vi "4.7.vi"() -> ()   [LabVIEW 2017]
panel:
  out "猜测次数":dbl
  out "随机的数":dbl
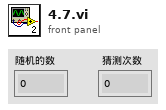
[diagram p1: front panel]
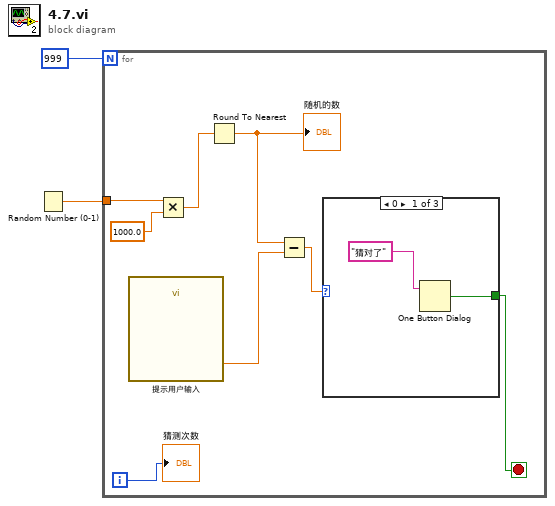
[diagram p0: block diagram]
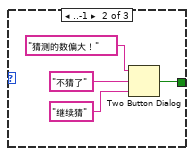
[diagram p2: hidden frame]
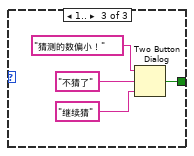
[diagram p3: hidden frame]
diagram:
  n1 = Random Number (0-1)() -> (number: 0 to 1=w1:dbl)
  n2 = for {
    N: 999 -> [_]
    tunnel: w1 -> [w3]
    i -> [w8]
    stop <- w4 stop-if-true
    n3 = call "提示用户输入"() -> ("请在1-1000猜"=w6:dbl)  [unwired: 17 in, 2 out]
    n4 = Multiply(x=w3, y=1000.0) -> (x*y=w9:dbl)
    n5 = Round To Nearest(number=w9) -> (nearest integer value=w7:dbl)
    "随机的数" <- w7
    n6 = Subtract(x=w7, y=w6) -> (x-y=w5:dbl)
    n7 = case shown="0" w5 {
      tunnel: [w11 w13 w17] -> w4
      frame 0 {
        n8 = One Button Dialog(message="猜对了") -> (true=w11:bool)  [unwired: 1 in]
      }
      frame ..-1 {
        n9 = Two Button Dialog(message="猜测的数偏大！", 1:"继续猜", 2:"不猜了") -> (T button?=w13:bool)
      }
      frame 1.. {
        n10 = Two Button Dialog(message="猜测的数偏小！", 1:"继续猜", 2:"不猜了") -> (T button?=w17:bool)
      }
    }
    "猜测次数" <- w8
  }
